vi "Initialize Hardware.vi"(8 "error in (no error)":errorcluster, 9 "Connection Setting":T1={"Connection Ref"=variant, "Serial Configuration"={"Baud Rate"=9600, "Parity"=2, "Data Bits"=7}} {"Serial Configuration"."Data Bits" items=["7"=7, "8"=8]; "Serial Configuration"."Parity" items=["None", "Odd", "Even"]; "Serial Configuration"."Baud Rate" items=["300"=300, "600"=600, "1200"=1200, "2400"=2400, "4800"=4800, "9600"=9600, "19200"=19200]}, 10 "DAQ Type":enum16{"Hardware", "Simulation"}(ring), 11 "Agilent 34401A in":refnum<class "Agilent 34401A.lvclass">) -> (0 "error out":errorcluster, 3 "Agilent 34401A out":refnum<class "Agilent 34401A.lvclass">)   [LabVIEW 2021, in "DMM.lvlib" / "Agilent 34401A.lvclass"]
uses:
  Agilent 34401A.lvclass
  Agilent 34401A.lvclass/Agilent 34401A.ctl
  <instrlib>/Agilent 34401/Agilent 34401.lvlib
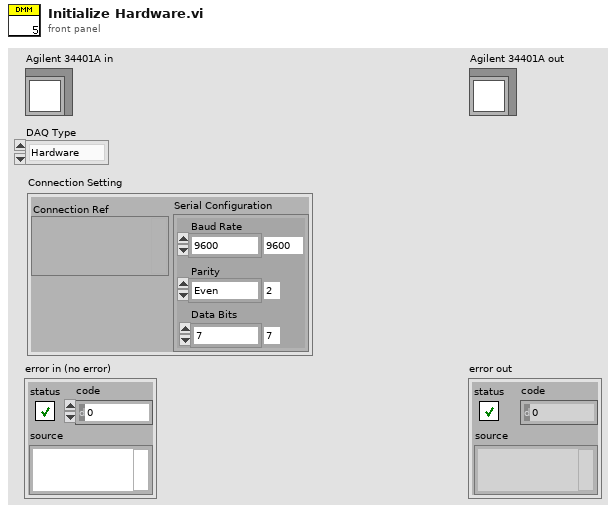
[diagram p1: front panel]
types:
  T1 = cluster{"Connection Ref":variant, "Serial Configuration":cluster{"Baud Rate":u32, "Parity":u16, "Data Bits":u16}}
  T2 = cluster{"Baud Rate":u32, "Parity":u16, "Data Bits":u16}
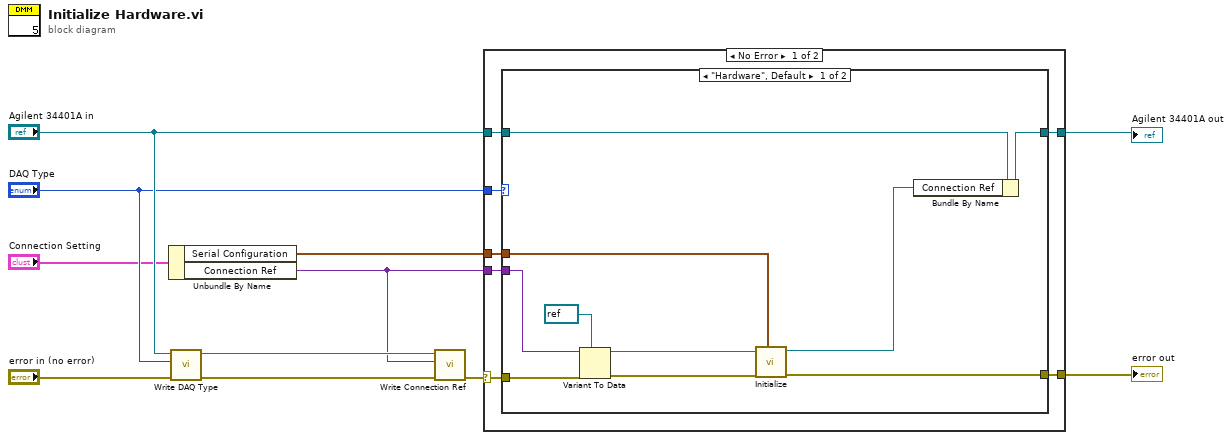
[diagram p0: block diagram]
diagram:
  n1 = Unbundle By Name("Connection Setting") -> ("Serial Configuration"=w2:T2, "Connection Ref"=w1:variant)
  n2 = call-dynamic "Write DAQ Type.vi"("error in (no error)"="error in (no error)", "DAQ Type"="DAQ Type", "Agilent 34401A in"="Agilent 34401A in") -> ("error out"=w10:errorcluster, "Agilent 34401A out"=w8:refnum<class "Agilent 34401A.lvclass">)  [unwired: 7 in]
  n3 = call-dynamic "Write Connection Ref.vi"("error in (no error)"=w10, "Connection Ref"=w1, "Agilent 34401A in"=w8) -> ("error out"=w9:errorcluster)  [unwired: 7 in, 1 out]
  n4 = case shown="No Error" w9 {
    selector: w9 -> [w17 w31]
    tunnel: "Agilent 34401A in" -> [w15 w32]
    tunnel: "DAQ Type" -> [w18 _]
    tunnel: [w16 w31] -> w5
    tunnel: [w14 w32] -> w4
    tunnel: w2 -> [w13 _]
    tunnel: w1 -> [w12 _]
    frame No Error {
      n5 = case shown="\"Hardware\", Default" w18 {
        tunnel: w17 -> [w28 w29]
        tunnel: [w24 w29] -> w16
        tunnel: w15 -> [w23 w30]
        tunnel: [w22 w30] -> w14
        tunnel: w13 -> [w20 _]
        tunnel: w12 -> [w19 _]
        frame "Hardware", Default {
          n6 = Variant To Data(error in=w28, type=refnum<visa-resource-name> refnum ("VISA resource name"), Variant=w19) -> (data=w26:refnum<visa-resource-name>, error out=w25:errorcluster)
          n7 = call <instrlib>:"Initialize.vi"("Serial Configuration"=w20, "error in (no error)"=w25, "VISA resource name"=w26) -> ("error out"=w24:errorcluster, "VISA resource name out"=w21:refnum<visa-resource-name>)  [unwired: 7 in]
          n8 = Bundle By Name(cluster=w23, "Connection Ref"=w21) -> (w22:refnum<class "Agilent 34401A.lvclass">)
        }
        frame "Simulation" {
        }
      }
    }
    frame Error {
    }
  }
  "error out" <- w5
  "Agilent 34401A out" <- w4
